vi "trusted client certfications.vi"(8 "Error In":errorcluster, 10 "OPC UA server refnum in":refnum<k21>, 11 "DOM document in":refnum<k20>) -> (0 "Error Out":errorcluster, 1 "trusted client certfications":path[](array[path]), 2 "OPC UA server refnum out":refnum<k21>, 3 "DOM document out":refnum<k20>)   [LabVIEW 2013, in "CreateOPCUAServerAuto.lvlib"]
uses:
  CreateOPCUAServerAuto.lvlib
  <vilib>/xml/Close Reference(Node).vi
  <resource>/objmgr/DOMUserDefRef.rc
  <vilib>/xml/NI_XML.lvlib
  <vilib>/OPCUA/NI OPC UA Server.lvlib
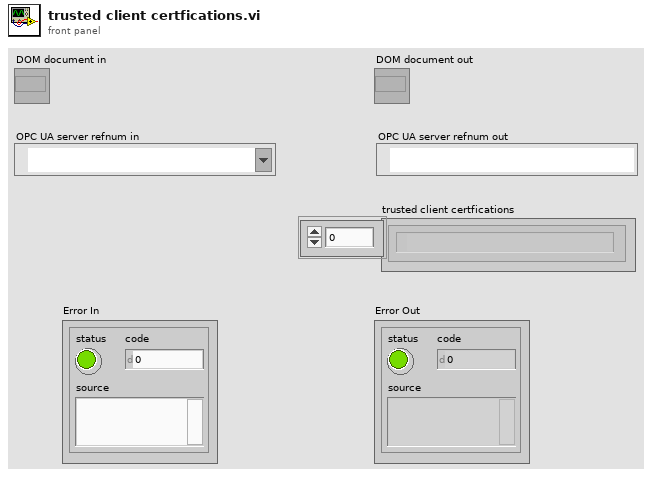
[diagram p1: front panel]
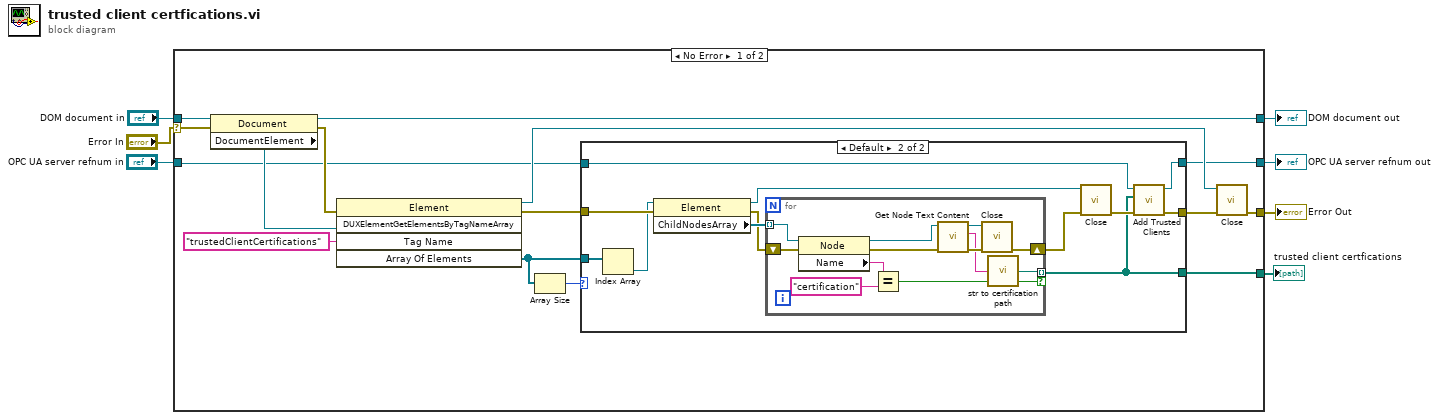
[diagram p0: block diagram]
diagram:
  n1 = case shown="No Error" "Error In" {
    selector: "Error In" -> [w22 w51]
    tunnel: [w19 w51] -> w7
    tunnel: "DOM document in" -> [w21 w50]
    tunnel: [w20 w50] -> w4
    tunnel: [w10 w49] -> w3
    tunnel: "OPC UA server refnum in" -> [w9 w49]
    tunnel: [w8 _] -> w1
    frame No Error {
      n2 = property class="Document"(reference=w21, error in=w22) -> (reference out=w20:refnum<k20>, error out=w14:errorcluster, "DocumentElement"=w16:refnum<k20>)
      n3 = invoke class="Element" method="DUXElementGetElementsByTagNameArray"(reference=w16, error in=w14, "Tag Name"="trustedClientCertifications") -> (reference out=w13:refnum<k20>, error out=w17:errorcluster, "Array Of Elements"=w12:refnum<k20>[])  [unwired: 2 in, 2 out]
      n4 = Array Size(array=w12) -> (size(s)=w11:i32)
      n5 = case shown="Default" w11 {
        tunnel: [w24 w28] -> w18
        tunnel: w17 -> [w24 w36]
        tunnel: w12 -> [_ w31]
        tunnel: [w23 w27] -> w10
        tunnel: w9 -> [w23 w26]
        tunnel: [_ w25] -> w8
        frame 0 {
        }
        frame Default {
          n6 = Index Array(array=w31) -> (element=w30:refnum<k20>)  [unwired: 1 in]
          n7 = property class="Element"(reference=w30, error in=w36) -> (reference out=w35:refnum<k20>, error out=w33:errorcluster, "ChildNodesArray"=w34:refnum<k20>[])
          n8 = for {
            tunnel: w34 -> [w45] mode=indexing
            tunnel: [w37] -> w25 mode=indexing if=w40
            shift-right: [w46] -> w32
            shift-left: w33 -> [w44]
            n9 = property class="Node"(reference=w45, error in=w44) -> (reference out=w43:refnum<k20>, error out=w39:errorcluster, "Name"=w42:string)
            n10 = Equal?(x=w42, y="certification") -> (x = y?=w40:bool)
            n11 = call <vilib>:"Get Node Text Content.vi"("error in (no error)"=w39, "node in"=w43) -> ("error out"=w48:errorcluster, "node text"=w38:string, "node out"=w47:refnum<k20>)  [unwired: 7 out]
            n12 = call-poly <vilib>:"Close.vi"("error in (no error)"=w48, "node"=w47) -> ("error out"=w46:errorcluster)  [unwired: 7 out]
            n13 = call "str to certification path.vi"("node text"=w38) -> ("File Path Control"=w37:path)  [unwired: 4 in]
          }
          n14 = call-poly <vilib>:"Close.vi"("error in (no error)"=w32, "node"=w35) -> ("error out"=w29:errorcluster)  [unwired: 7 out]
          n15 = call <vilib>:"Add Trusted Clients.vi"("error in (no error)"=w29, "trusted client certificates"=w25, "OPC UA server refnum in"=w26) -> ("error out"=w28:errorcluster, "OPC UA server refnum out"=w27:refnum<k21>)  [unwired: 7 in]
        }
      }
      n16 = call-poly <vilib>:"Close.vi"("error in (no error)"=w18, "node"=w13) -> ("error out"=w19:errorcluster)  [unwired: 7 out]
    }
    frame Error {
    }
  }
  "Error Out" <- w7
  "DOM document out" <- w4
  "OPC UA server refnum out" <- w3
  "trusted client certfications" <- w1
